vi "View.vi"(8 "error in (no error)":errorcluster, 10 "Ref for Sizing":refnum<vi>, 11 "Plot ID":T1 format="%x") -> (0 "error out":errorcluster, 2 "Picture":picture, 3 "Plot ID Out":T1 format="%x")   [LabVIEW 2013, in "Advanced Plotting Toolkit.lvlib"]
doc: "Render a plot as a LabView Picture."
uses:
  Advanced Plotting Toolkit.lvlib
  typedefs/PlotID.ctl
  <vilib>/picture/picture.llb/Draw True-Color Pixmap.vi
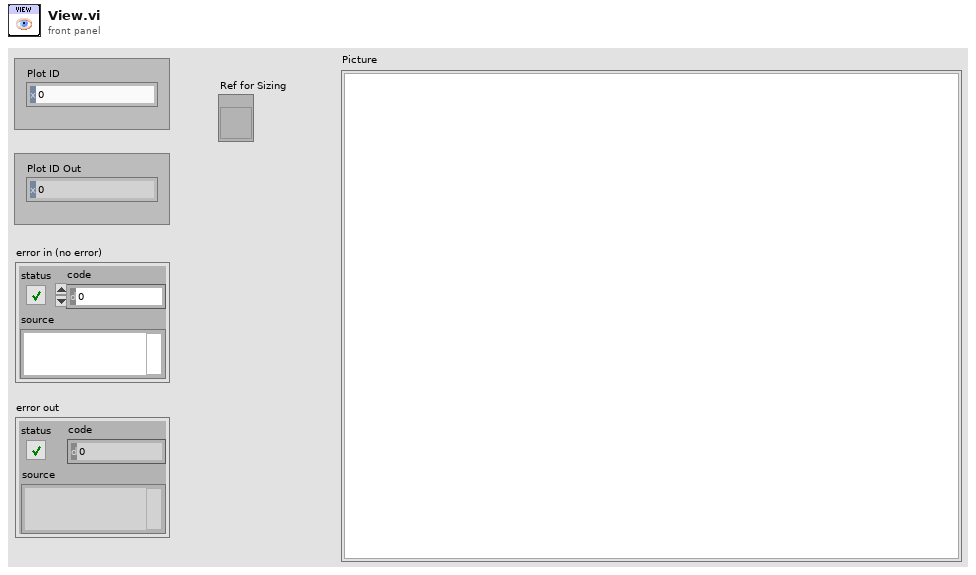
[diagram p1: front panel]
types:
  T1 = typedef "Advanced Plotting Toolkit.lvlib/PlotID.ctl" = i32
  T2 = enum16{"big-endian, network order", "native, host order", "little-endian"}
  T3 = typedef "Advanced Plotting Toolkit.lvlib/KeyValue.ctl" = cluster{"Key":string, "Value":string}
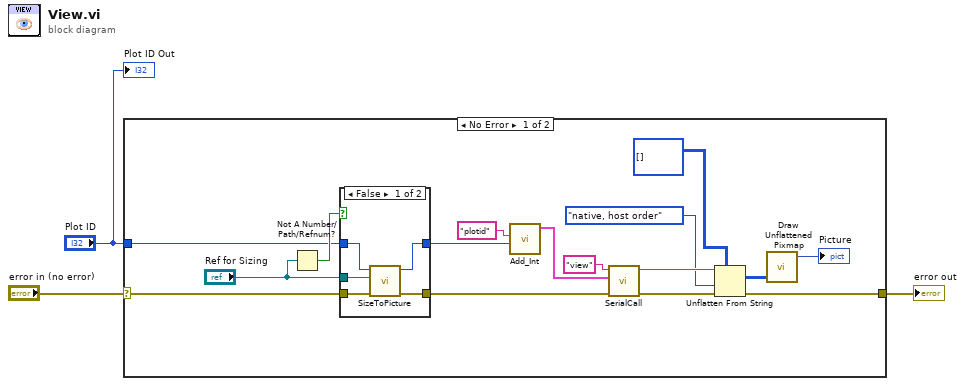
[diagram p0: block diagram]
diagram:
  n1 = case shown="No Error" "error in (no error)" {
    selector: "error in (no error)" -> [w18 w27]
    tunnel: [w4 w27] -> w3
    tunnel: "Plot ID" -> [w17 _]
    frame No Error {
      n2 = Not A Number/Path/Refnum?(number/path/refnum="Ref for Sizing") -> (NaN/Path/Refnum?=w19:bool)
      n3 = case shown="False" w19 {
        tunnel: w18 -> [w22 w26]
        tunnel: [w20 w26] -> w12
        tunnel: w17 -> [w24 w25]
        tunnel: [w21 w25] -> w11
        tunnel: "Ref for Sizing" -> [w23 _]
        frame False {
          n4 = call "SizeToPicture.vi"("error in (no error)"=w22, "Picture Reference"=w23, "Plot ID"=w24) -> ("error out"=w20:errorcluster, "Plot ID Out"=w21:T1)  [unwired: 7 in]
        }
        frame True {
        }
      }
      n5 = call "Add_Int.vi"("Value"=w11, "Key"="plotid") -> ("Keyword Array Out"=w13:T3[])  [unwired: 9 in]
      n6 = call "SerialCall.vi"("error in (no error)"=w12, "data"=w13, "Resource"="view") -> ("error out"=w5:errorcluster, "Response"=w10:string)  [unwired: 7 in]
      n7 = Unflatten From String(type=u32[][] [], binary string=w10, byte order (0:big-endian, network order)=T2."native, host order", error in (no error)=w5) -> (value=w8:u32[][], error out=w4:errorcluster)  [unwired: 1 in, 1 out]
      n8 = call-poly <vilib>:"Draw Unflattened Pixmap.vi"("data (RGB format)"=w8) -> ("new picture"=→"Picture":picture)  [unwired: 8 in]
    }
    frame Error {
    }
  }
  "error out" <- w3
  "Plot ID Out" <- "Plot ID"
